vi "Read TBD file.vi"(11 "文件路径（使用对话框）":path) -> (0 "末包数据量":i32, 1 "数据字符串":string, 2 "数组":string[](array[string]), 3 "数据包数":i32)   [LabVIEW 2013]
panel:
  out "替换数量":i32
  out "长度":i32
  out "结果字符串":string
  out "文本":string
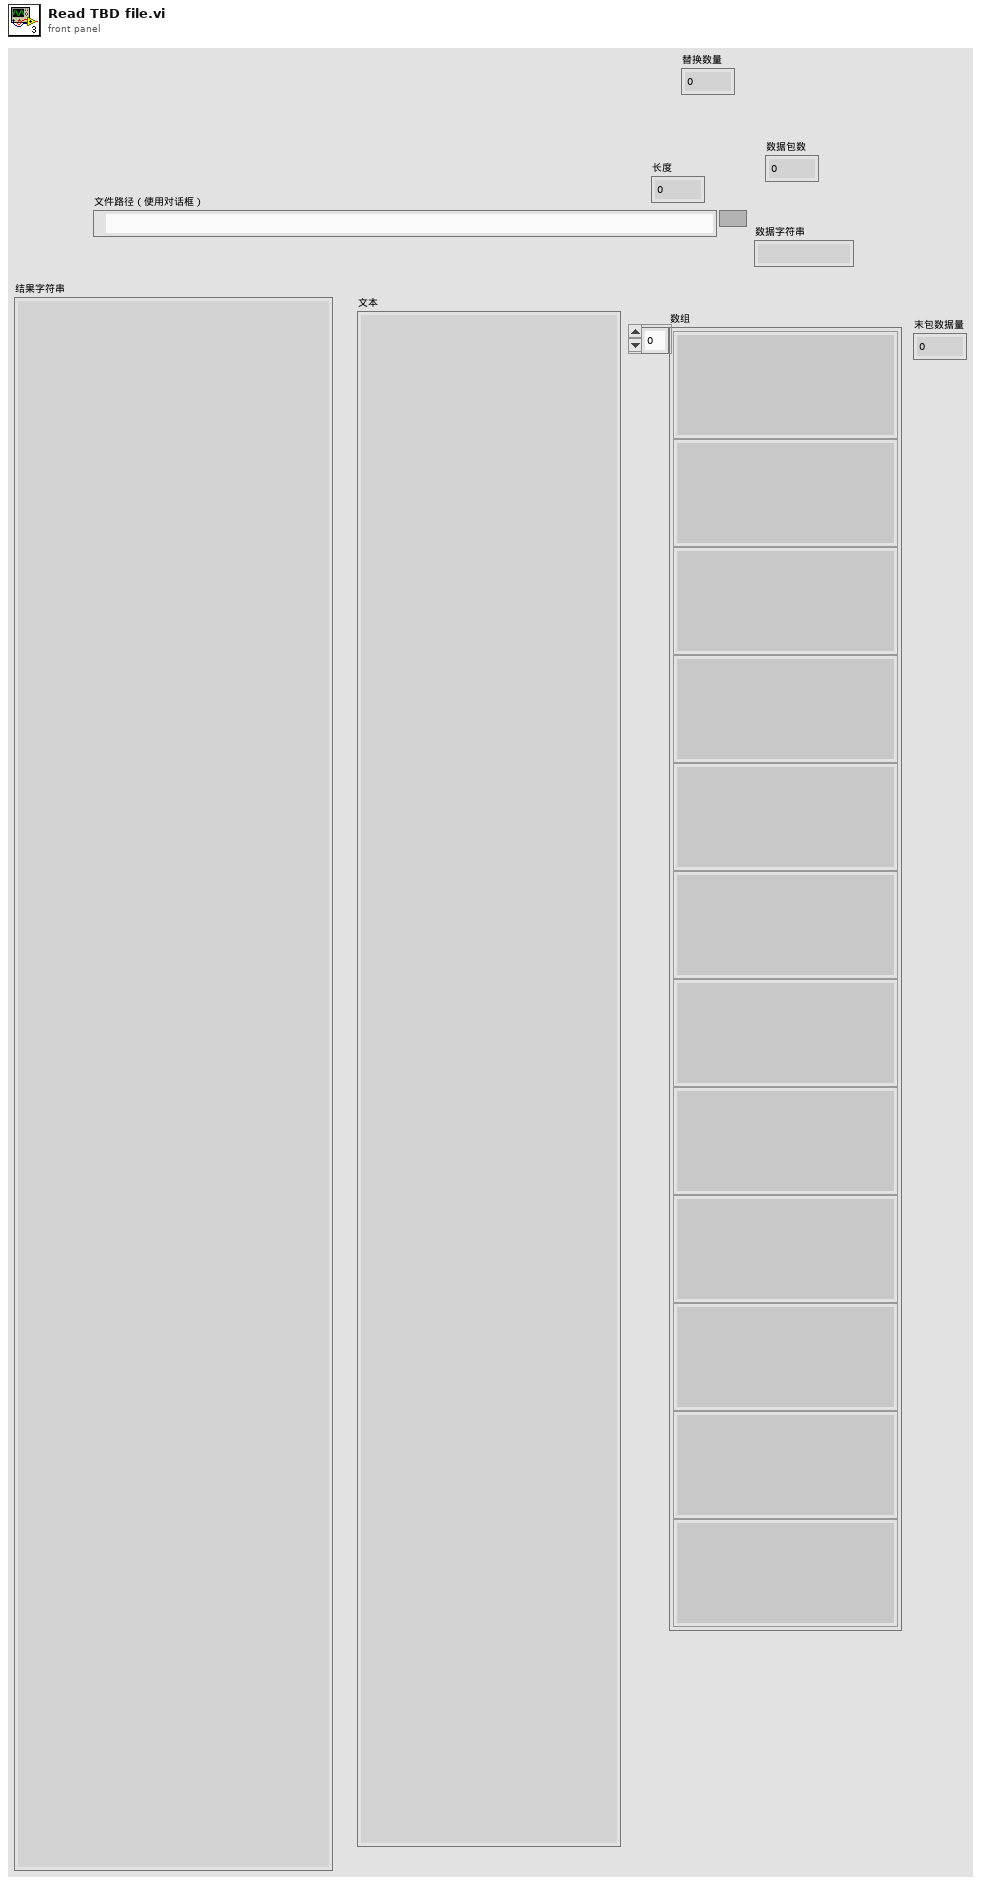
[diagram p1: front panel]
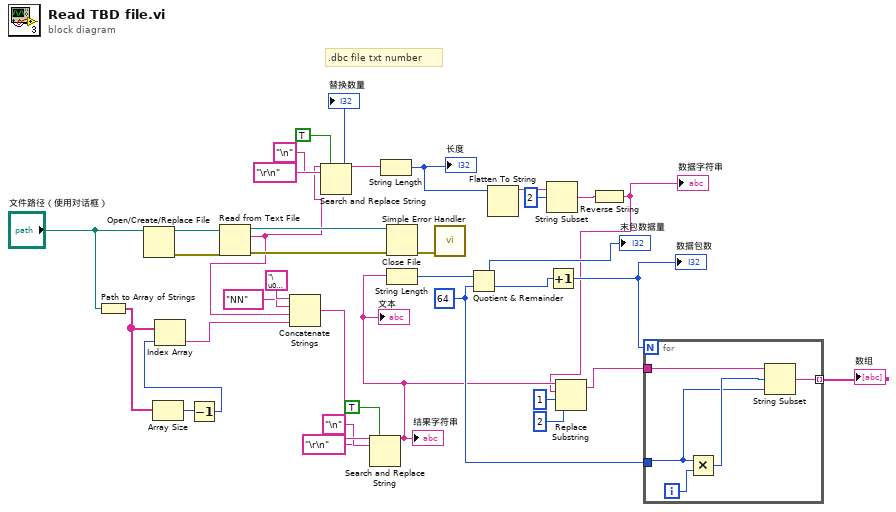
[diagram p0: block diagram]
diagram:
  w32 = 64 ("y")
  # ".dbc file txt number"
  n1 = Path to Array of Strings(0:"文件路径（使用对话框）") -> (2:w27:string[])  [unwired: 1 out]
  n2 = Open/Create/Replace File(file path (use dialog)="文件路径（使用对话框）") -> (refnum out=w37:refnum<file>, error out=w36:errorcluster)  [unwired: 5 in, 1 out]
  n3 = Array Size(array=w27) -> (size(s)=w26:i32)
  n4 = Decrement(x=w26) -> (x-1=w25:i32)
  n5 = Index Array(array=w27, index=w25) -> (element=w21:string)
  n6 = Read from Text File(file (use dialog)=w37, error in=w36) -> (refnum out=w34:refnum<file>, text=w5:string, error out=w35:errorcluster)  [unwired: 2 in, 1 out]
  n7 = Concatenate Strings("\u0002", "NN" ("字符串"), w5, w21) -> (w15:string)
  n8 = Search and Replace String(replace all?=TRUE ("替换全部？(F)"), input string=w5, search string="\n" ("搜索字符串"), replace string="\r\n" ("替换字符串(\"\")")) -> (result string=w7:string, number of replacements=→"替换数量":i32)  [unwired: 4 in, 2 out]
  n9 = Search and Replace String(replace all?=TRUE ("替换全部？(F)"), input string=w15, search string="\n" ("搜索字符串"), replace string="\r\n" ("替换字符串(\"\")")) -> (result string=w11:string)  [unwired: 4 in, 3 out]
  "文本" <- w11
  "结果字符串" <- w11
  n10 = String Length(string=w7) -> (length=w6:i32)
  "长度" <- w6
  n11 = Close File(refnum=w34, error in=w35) -> (error out=w1:errorcluster)  [unwired: 1 out]
  n12 = String Length(string=w11) -> (length=w24:i32)
  n13 = call <vilib>:"Simple Error Handler.vi"("error in (no error)"=w1) -> ()  [unwired: 4 in, 5 out]
  n14 = Quotient & Remainder(x=w24, y=w32) -> (x-y*floor(x/y)=→"末包数据量":i32, floor(x/y)=w30:i32)
  n15 = Flatten To String(anything=w6) -> (data string=w23:string)  [unwired: 3 in, 2 out]
  n16 = String Subset(string=w23, offset (0)=2 ("偏移量(0)")) -> (substring=w3:string)  [unwired: 1 in]
  n17 = Increment(x=w30) -> (x+1=w33:i32)
  "数据包数" <- w33
  n18 = Reverse String(1:w3) -> (0:w2:string)
  "数据字符串" <- w2
  n19 = Replace Substring(2:2 ("长度（子字符串长度）"), 3:1 ("偏移量(0)"), 4:w2, 5:w11) -> (1:w18:string)  [unwired: 1 out]
  n20 = for {
    N: w33 -> [_]
    tunnel: w18 -> [w42]
    tunnel: w32 -> [w39]
    tunnel: [w38] -> w31 mode=indexing
    i -> [w41]
    n21 = Multiply(x=w39, y=w41) -> (x*y=w40:i32)
    n22 = String Subset(string=w42, offset (0)=w40, length (rest)=w39) -> (substring=w38:string)
  }
  "数组" <- w31
